vi "Get Common Root Folder.vi"(8 "Error In":errorcluster, 11 "Array of File Paths":path[](array[path])) -> (0 "Error Out":errorcluster, 3 "Common Folder Path":path)   [LabVIEW 2021, in "Files.lvlib"]
uses:
  Files.lvlib
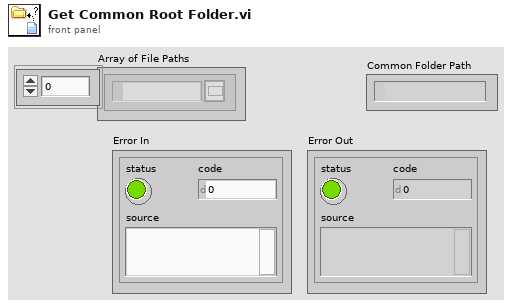
[diagram p1: front panel]
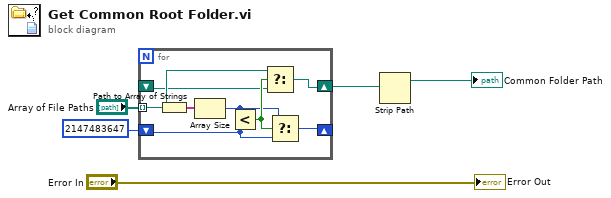
[diagram p0: block diagram]
diagram:
  n1 = for {
    tunnel: "Array of File Paths" -> [w7] mode=indexing
    shift-right: [w8] -> _
    shift-left: 2147483647 ("size(s)") -> [w9]
    shift-right: [w12] -> w2
    shift-left: _ -> [w6]
    n2 = Path to Array of Strings(0:w7) -> (2:w13:string[])  [unwired: 1 out]
    n3 = Array Size(array=w13) -> (size(s)=w10:i32)
    n4 = Less?(x=w10, y=w9) -> (x < y?=w11:bool)
    n5 = Select(t=w7, s=w11, f=w6) -> (s? t:f=w12:path)
    n6 = Select(t=w10, s=w11, f=w9) -> (s? t:f=w8:i32)
  }
  n7 = Strip Path(path=w2) -> (stripped path=→"Common Folder Path":path)  [unwired: 1 out]
  "Error Out" <- "Error In"
